vi "Read DMA and Update Waveform.vi"(4 "Delacing Scheme":T2, 6 "Number of Channels":u8, 7 "Timeout?":bool, 8 "error in (no error)":errorcluster, 9 "Total Samples":u32, 10 "DMA Ref":T1, 11 "Multiple Waveforms Write (DBL) in":refnum<class "Multiple Waveforms Write (DBL).lvclass">) -> (0 "error out":errorcluster, 1 "Elements Remaining":u32, 2 "FPGA VI Reference Out":T1, 3 "Multiple Waveforms Write (DBL) out":refnum<class "Multiple Waveforms Write (DBL).lvclass">)   [LabVIEW 2016, in "FPGA Addon Engine.lvlib"]
uses:
  FPGA Addon Engine.lvlib
  Shared/Delacing Scheme.ctl
  Types/DMA Input Ref.ctl
  <vilib>/NI Veristand/Custom Device Waveform API/Multiple Waveforms Write (DBL)/Multiple Waveforms Write (DBL).lvclass
  C:/Program Files (x86)/National Instruments/LabVIEW 2016/vi.lib/NI Veristand/Custom Device Waveform API/Waveform Session.lvclass
  <vilib>/NI Veristand/Custom Device Waveform API/Waveform Session.lvclass/Waveform Session.ctl
  <vilib>/NI Veristand/Custom Device Waveform API/Multiple Waveforms Write (DBL)/Multiple Waveforms Write (DBL).lvclass/Multiple Waveforms Write (DBL).ctl
  <vilib>/NI Veristand/Custom Device Waveform API/Internal Comm Classes/WPL Comm/WPL Comm (2D DBL)/WPL Comm (2D DBL).lvclass/WPL Comm (2D DBL).ctl
  <vilib>/NI Veristand/Custom Device Waveform API/Internal Comm Classes/WPL Comm/WPL Comm.lvclass/WPL Comm.ctl
  <vilib>/NI Veristand/Custom Device Waveform API/Multiple Waveforms Write (DBL)/NI VeriStand - Write Multiple Waveforms (DBL).vi
  <vilib>/NI Veristand/Custom Device Waveform API/Read Sample offset DVR.vi
  <vilib>/NI Veristand/Custom Device Waveform API/Internal Comm Classes/WPL Comm/WPL Comm (2D DBL)/Comm_write 2d dbl.vi
  <vilib>/NI Veristand/Custom Device Waveform API/Check Write Size.vi
  <vilib>/NI Veristand/Custom Device Waveform API/Check Opened.vi
  <vilib>/NI Veristand/Custom Device Waveform API/Internal Comm Classes/WPL Comm/Direct Send WPL Command.vi
  <vilib>/NI Veristand/Custom Device Waveform API/Internal Comm Classes/WPL Comm/Convert Q Error to Shutdown Error.vi
  <vilib>/NI Veristand/Custom Device Waveform API/Internal Comm Classes/WPL Comm/WPL Comm (2D DBL)/WPL Comm (2D DBL).lvclass
  C:/Program Files (x86)/National Instruments/LabVIEW 2016/vi.lib/NI Veristand/Custom Device Waveform API/Internal Comm Classes/WPL Comm/WPL Comm.lvclass
  <vilib>/Utility/error.llb/Error Cluster From Error Code.vi
  <vilib>/rvi/errors/niLvFpgaAdjustHostInterfaceError.vi
  <vilib>/rvi/interface/nirviMethod/nirviMethod.xnode
  <vilib>/NI VeriStand/Custom Device Waveform API/NI_VS Custom Device Waveform API.lvlib
  <vilib>/FPGAPlugInAG/Dynamic/niLvFpga_ReadFifo_Dynamic.vi
  <vilib>/rvi/errors/niLvFpgaMergeErrorWithErrorCode.vi
  Shared/FPGA Addon Shared.lvlib
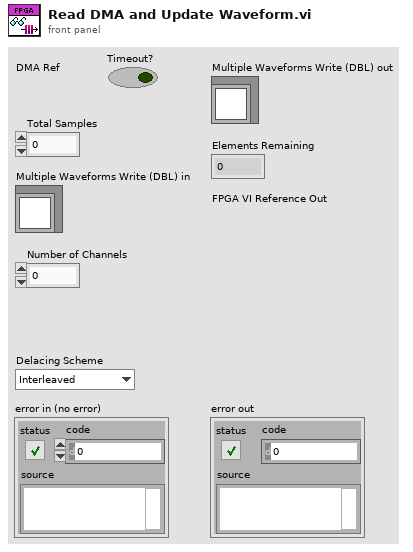
[diagram p1: front panel]
types:
  T1 = typedef "FPGA Addon Engine.lvlib/DMA Input Ref.ctl" = refnum<k20>
  T2 = typedef "FPGA Addon Shared.lvlib/Delacing Scheme.ctl" = enum8{"Interleaved"}
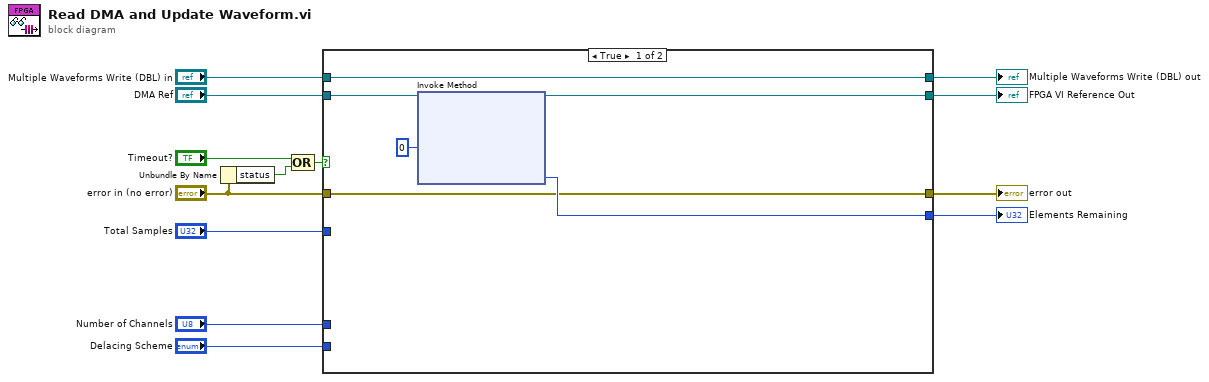
[diagram p0: block diagram]
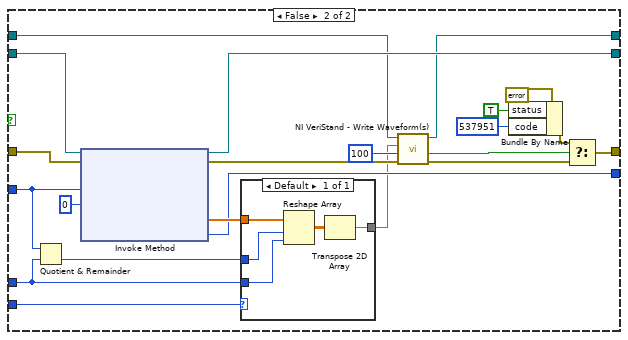
[diagram p2: hidden frame]
diagram:
  n1 = Unbundle By Name("error in (no error)") -> ("status"=w3:bool)
  n2 = Compound Arithmetic op=OR("Timeout?", w3) -> (w1:bool)
  n3 = case shown="True" w1 {
    tunnel: [w14 w40] -> w13
    tunnel: [w15 w33] -> w12
    tunnel: "Delacing Scheme" -> [_ w31]
    tunnel: [w17 w30] -> w10
    tunnel: "DMA Ref" -> [w18 w29]
    tunnel: [w19 w28] -> w8
    tunnel: "Multiple Waveforms Write (DBL) in" -> [w19 w24]
    tunnel: "Total Samples" -> [_ w23]
    tunnel: "Number of Channels" -> [_ w22]
    tunnel: "error in (no error)" -> [w14 w20]
    frame True {
      w16 = 0 ("Timeout (ms)")
      n4 = xnode "Invoke Method"("FPGA VI Reference In"=w18, "Number of Elements"=w16, "Timeout (ms)"=w16) -> ("FPGA VI Reference Out"=w17:T1, "Elements Remaining"=w15:u32)  [unwired: 1 in, 2 out]
    }
    frame False {
      n5 = Quotient & Remainder(x=w23, y=w22) -> (floor(x/y)=w21:u32)  [unwired: 1 out]
      n6 = xnode "Invoke Method"("FPGA VI Reference In"=w29, "error in"=w20, "Number of Elements"=w23, "Timeout (ms)"=0) -> ("FPGA VI Reference Out"=w30:T1, "error out"=w27:errorcluster, "Data"=w41:sgl[], "Elements Remaining"=w33:u32)
      n7 = case shown="Default" w31 {
        tunnel: w41 -> [w45]
        tunnel: [w44] -> w26
        tunnel: w22 -> [w43]
        tunnel: w21 -> [w42]
        frame Default {
          n8 = Reshape Array(w45, w42, w43) -> (w46:sgl[][])
          n9 = Transpose 2D Array(2D array=w46) -> (transposed array=w44:sgl[][])
        }
      }
      n10 = call-poly <vilib>:"NI VeriStand - Write Waveform(s).vi"("error in (no error)"=w27, "timeout in ms (0)"=100, "Data"=w26, "Multiple Waveforms Write Session (DBL) in"=w24) -> ("error out"=w39:errorcluster, "timed out?"=w34:bool, "Multiple Waveforms Write Session (DBL) out"=w28:refnum<class "Multiple Waveforms Write (DBL).lvclass">)  [unwired: 5 in]
      n11 = Bundle By Name(cluster=errorcluster {"status"=FALSE, "code"=0, "source"=""} ("input cluster"), "status"=TRUE, "code"=537951) -> (w38:errorcluster)
      n12 = Select(t=w38, s=w34, f=w39) -> (s? t:f=w40:errorcluster)
    }
  }
  "error out" <- w13
  "Elements Remaining" <- w12
  "FPGA VI Reference Out" <- w10
  "Multiple Waveforms Write (DBL) out" <- w8
